vi "TEST_ASIC_SUMnADDS.vi"(0 "Instrument VISA in":T1={"AWG VISA"="generadorpulsos", "Oscilloscope  VISA "="Oscilloscope", "Integration Board IP"="172.16.7.43", "connection ID"=refnum, "report out"=refnum, "report file path"=path "C:/Documents and Settings/CTA_LAB01/Desktop/L0_Asic/L0 Asic Test Data"}, 2 "Serial number":string="SN018", 5 "quantity":i32=3, 7 "Cycles Burst":i32=10000, 9 "L1 Address":i32=17, 11 "error in":errorcluster, 12 "channel array":i32[](array[numeric])=[0, 1, 2, 3, 4, 5, 6]) -> (4 "Instrument VISA out":T1={"AWG VISA"="", "Oscilloscope  VISA "="", "Integration Board IP"="", "connection ID"=refnum, "report out"=refnum, "report file path"=path "C:/Documents and Settings/CTA_LAB01/Desktop/L0_Asic/L0 Asic Test Data"}, 15 "error out":errorcluster={"status"=TRUE, "code"=63, "source"="TCP Open Connection in Test2_3b_ASIC_mezzanine.vi->test_sum_mezzanine_ASIC.vi"})   [LabVIEW 2009]
uses:
  <vilib>/Utility/NIReport.llb/NI_report.lvclass
  <vilib>/Utility/NIReport.llb/HTML/NI_HTML.lvclass
  <instrlib>/Agilent 81150/Agilent 81150.lvlib
  <instrlib>/Agilent 8000 Series/Agilent 8000 Series.lvlib
panel:
  out "NChannels":i32
  out "Array":i32[](array[numeric])=[0, 2, 3]
  out "Filename Out":path
  out "points quantity":dbl=138.0
  out "appended array":dbl[](array[numeric])=[0.05, 11.0, 0.0, 63.0, 1.0, 9.99999e+37, 9.99999e+37, 2.068e-09, 3.4e-11, 9.99999e+37, 9.99999e+37, 9.99999e+37, 9.99999e+37, 9.99999e+37, 9.99999e+37, 138.0]
  out "read buffer 3":string="V amptd(1),9.99999E+37,9.99999E+37,9.99999E+37,9.99999E+37,9.99999E+37,1.38E+02,+ width(1),2.06E-09,1.99E-09,2.19E-09,2.068E-09,3.4E-11,1.38E+02,V amptd(f2),9.99999E+37,9.99999E+37,9.99999E+37,9.99999E+37,9.99999E+37,1.38E+02,+ width(f2),9.99999E+37,9.99999E+37,9.99999E+37,9.99999E+37,9.99999E+37,3.5E+01,Time(1-f2),9.99999E+37,9.99999E+37,9.99999E+37,9.99999E+37,9.99999E+37,1.00E+02\n"
  in  "Quantity of \nMeasurements":u32=50
  in  "Voltage":dbl[](array[numeric])=[0.05, 0.2]
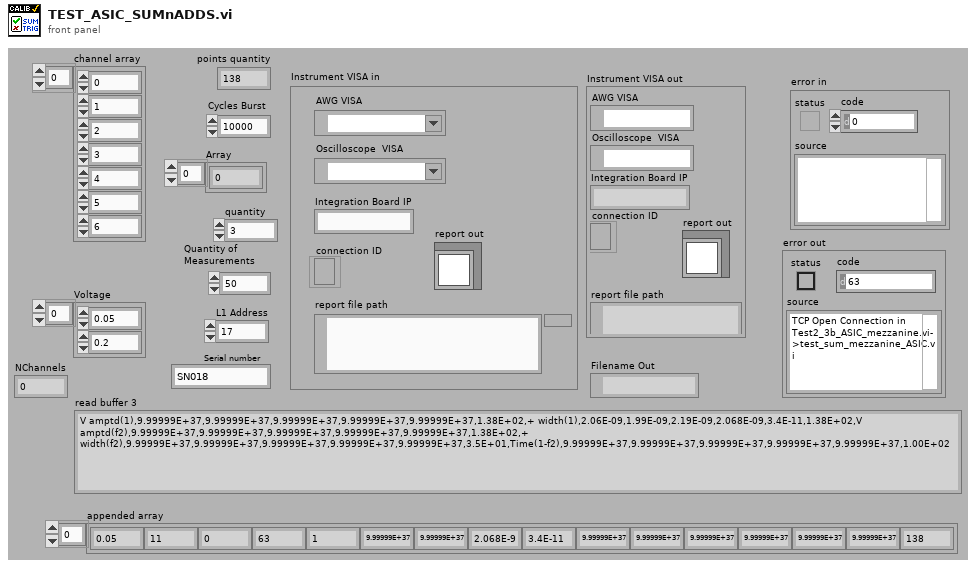
[diagram p1: front panel]
types:
  T1 = cluster{"AWG VISA":refnum<visa-resource-name>, "Oscilloscope  VISA ":refnum<visa-resource-name>, "Integration Board IP":string, "connection ID":refnum<k5>, "report out":refnum<class "NI_report.lvclass">, "report file path":path}
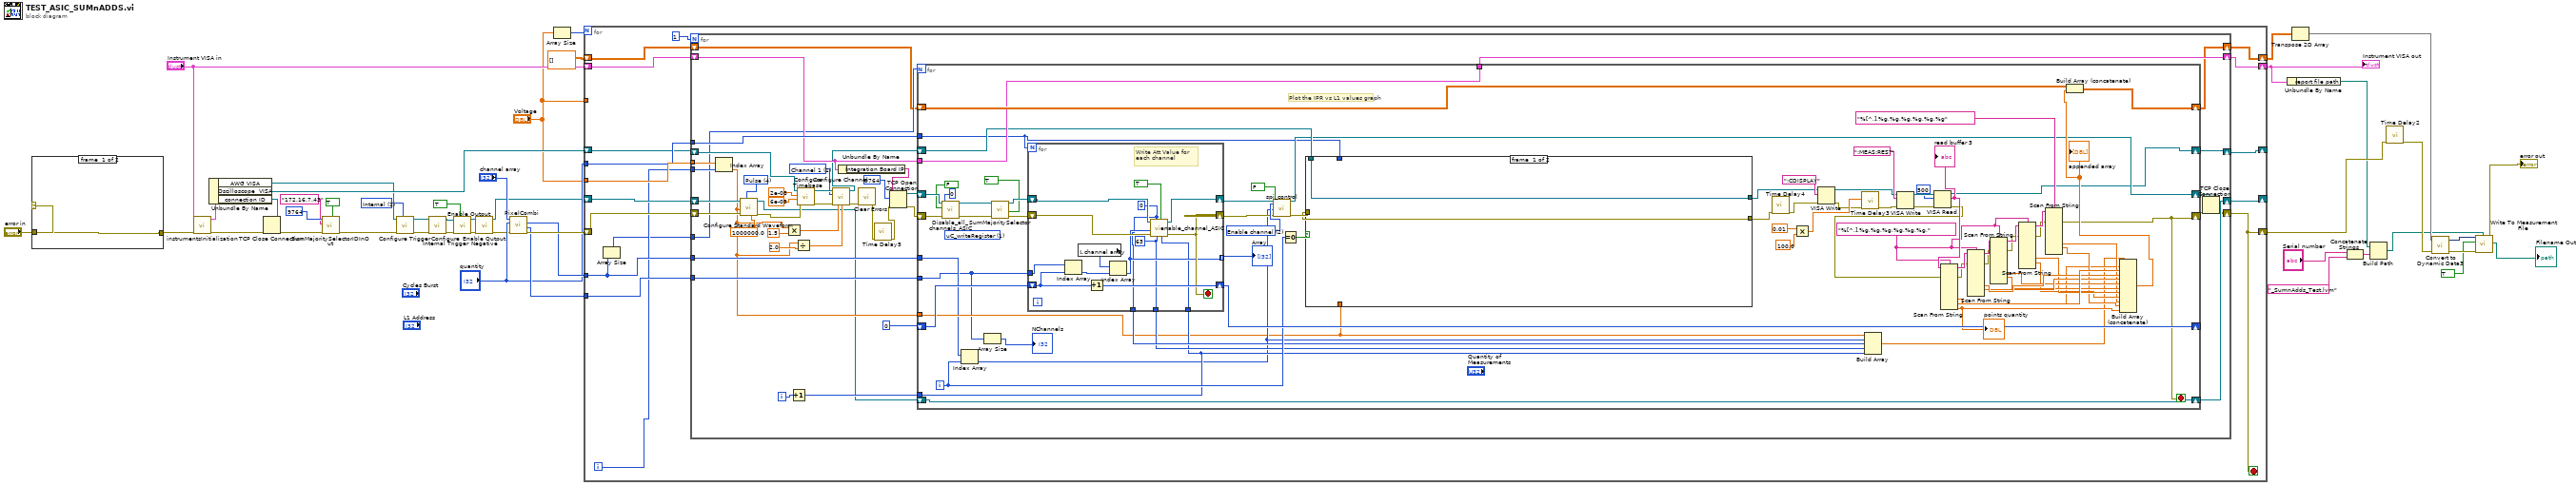
[diagram p0: block diagram]
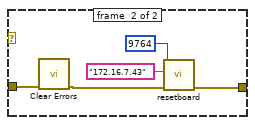
[diagram p2: hidden frame]
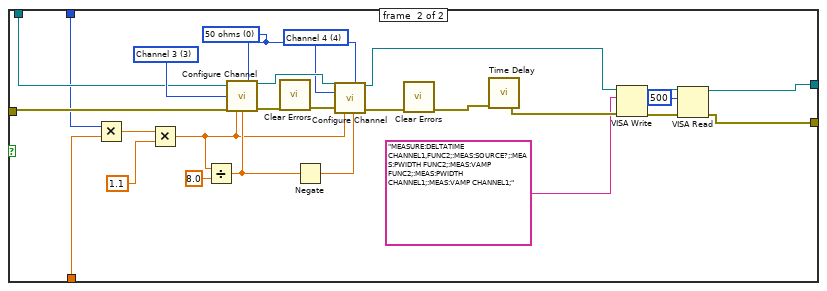
[diagram p3: hidden frame]
diagram:
  w22 = u16 1 items=["Immediate", "Internal", "External", "Software Trigger Function"] ("Trigger Source (0: Immediate)")
  n1 = case shown="Error" "error in" {
    tunnel: "error in" -> [w46 w48]
    tunnel: [w46 w51] -> w18
    frame #0 {
    }
    frame #1 {
      n2 = call <vilib>:"Clear Errors.vi"("error in (no error)"=w48) -> ("error out"=w47:errorcluster)  [unwired: 6 in]
      n3 = call "resetboard.vi"("error in (no error)"=w47, "address"="172.16.7.43", "remote port or service name"=u16 9764) -> ("error out"=w51:errorcluster)  [unwired: 7 in, 1 out]
    }
  }
  n4 = call "instrumentsInitialization.vi"("error in"=w18, "Instrument VISA in"="Instrument VISA in") -> ("error out"=w16:errorcluster, "Instrument VISA out"=w38:T1)  [unwired: 8 in]
  n5 = Unbundle By Name(w38) -> ("AWG VISA"=w25:refnum<visa-resource-name>, "Oscilloscope  VISA"=w37:refnum<visa-resource-name>, "connection ID"=w17:refnum<k5>)
  n6 = TCP Close Connection(connection ID=w17, error in (no error)=w16) -> (error out=w5:errorcluster)  [unwired: 1 in, 1 out]
  n7 = call "SumMajoritySelectorIDInOut.vi"("On Sum\nOff Majority"=TRUE ("Enable Output (T: Enable)"), "error in (no error)"=w5, "address"="172.16.7.43", "remote port or service name"=u16 9764) -> ("error out"=w1:errorcluster)  [unwired: 7 in]
  n8 = call <instrlib>:"Configure Trigger.vi"("Trigger Source (0: Immediate)"=w22, "error in (no error)"=w1, "VISA resource name"=w25) -> ("error out"=w23:errorcluster, "VISA resource name out"=w24:refnum<visa-resource-name>)  [unwired: 7 in]
  n9 = call <instrlib>:"Configure Internal Trigger.vi"("error in (no error)"=w23, "VISA resource name"=w24) -> ("error out"=w26:errorcluster, "VISA resource name out"=w27:refnum<visa-resource-name>)  [unwired: 8 in]
  n10 = call <instrlib>:"Enable Output.vi"("Enable Output (T: Enable)"=TRUE, "error in (no error)"=w26, "VISA resource name"=w27) -> ("error out"=w13:errorcluster, "VISA resource name out"=w12:refnum<visa-resource-name>)  [unwired: 7 in]
  n11 = call <instrlib>:"Enable Output Negative.vi"("error in (no error)"=w13, "VISA resource name"=w12) -> ("error out"=w14:errorcluster, "VISA resource name out"=w15:refnum<visa-resource-name>)  [unwired: 8 in]
  n12 = call "PixelCombi.vi"("error in"=w14, "quantity"="quantity", "array"="channel array") -> ("error out"=w44:errorcluster, "Channels"=w43:i32[], "Combination Array"=w42:i16[])  [unwired: 6 in]
  n13 = Array Size(array="Voltage") -> (size(s)=w39:i32)
  n14 = for {
    N: w39 -> [_]
    tunnel: w43 -> [w66]
    tunnel: w42 -> [w65]
    shift-right: [w52] -> w29
    shift-left: w44 -> [w68]
    tunnel: "Voltage" -> [w64]
    tunnel: "Voltage" -> [_]
    tunnel: "quantity" -> [w62]
    shift-right: [w57] -> w28
    shift-left: "Instrument VISA in" -> [w60]
    shift-right: [w56] -> w32
    shift-left: dbl[][] [] -> [w58]
    shift-right: [w53] -> _
    shift-left: w15 -> [w67]
    shift-right: [w54] -> _
    shift-left: w37 -> [w61]
    i -> [w63]
    stop <- w52 stop-if-true
    n15 = Array Size(array=w65) -> (size(s)=w59:i32)
    n16 = for {
      N: 1 -> [_]
      tunnel: w66 -> [w107]
      tunnel: w65 -> [w105]
      tunnel: w64 -> [w104]
      tunnel: w63 -> [w103]
      tunnel: w62 -> [w102]
      tunnel: w59 -> [w87]
      shift-right: [w77] -> w56
      shift-left: w58 -> [w80]
      shift-right: [w78] -> w57
      shift-left: w60 -> [w91]
      shift-right: [w72] -> w52
      shift-left: w68 -> [w109]
      shift-right: [w73] -> w53
      shift-left: w67 -> [w108]
      shift-right: [w75] -> w54
      shift-left: w61 -> [w98]
      i -> [w69]
      w94 = 1 items=["Channel 1"=1, "Channel 2"=2, "Channel 3"=3, "Channel 4"=4] ("Channel (1: Channel 1)")
      w111 = u16 4 items=["Sine", "Square", "Ramp Up", "Ramp Down", "Pulse", "Noise", "DC"] ("Waveform (0: Sine)")
      n17 = Index Array(array=w104, index=w103) -> (element=w79:dbl)
      n18 = call <instrlib>:"Configure Standard Waveform.vi"("Frequency (1000.0 Hz)"=1000000.0, "Waveform (0: Sine)"=w111, "error in (no error)"=w109, "Amplitude (1.0 Vpp)"=w79, "VISA resource name"=w108) -> ("error out"=w101:errorcluster, "VISA resource name out"=w74:refnum<visa-resource-name>)  [unwired: 5 in]
      n19 = Multiply(x=w79, y=1.5) -> (x*y=w93:dbl)
      n20 = Increment(x=w69) -> (x+1=w76:i32)
      n21 = Divide(x=w79, y=2.0) -> (x/y=w85:dbl)
      n22 = call <instrlib>:"Configure Timebase.vi"("error in (no error)"=w101, "Position (0.0 s)"=6e-09, "Timebase (0.005 s)"=2e-08, "VISA resource name"=w98) -> ("error out"=w100:errorcluster, "VISA resource name out"=w97:refnum<visa-resource-name>)  [unwired: 6 in]
      n23 = call <instrlib>:"Configure Channel.vi"("VISA resource name"=w97, "Channel (1: Channel 1)"=w94, "error in (no error)"=w100, "Vertical Range (2.0 V)"=w93, "Vertical Offset (0.0 V)"=w85) -> ("VISA resource name out"=w84:refnum<visa-resource-name>, "error out"=w99:errorcluster)  [unwired: 9 in]
      n24 = Unbundle By Name(w91) -> ("Integration Board IP"=w89:string)
      n25 = call <vilib>:"Clear Errors.vi"("error in (no error)"=w99) -> ("error out"=w71:errorcluster)  [unwired: 6 in]
      n26 = call "Time Delay5"("error in (no error)"=w71) -> ("error out"=w70:errorcluster)  [unwired: 10 in]
      n27 = TCP Open Connection(address=w89, remote port or service name=u16 9764, error in (no error)=w70) -> (connection ID=w81:refnum<k5>, error out=w90:errorcluster)  [unwired: 2 in]
      n28 = for {
        N: w87 -> [_]
        tunnel: w105 -> [w115]
        tunnel: w107 -> [w113]
        shift-right: [w185] -> _
        shift-left: i16 0 ("element") -> [w186]
        shift-right: [w135] -> w83
        shift-left: w90 -> [w181]
        tunnel: w91 -> [w176]
        tunnel: w102 -> [w112]
        tunnel: [w176] -> w78
        shift-right: [w182] -> w77
        shift-left: w80 -> [w183]
        shift-right: [w136] -> w82
        shift-left: w81 -> [w134]
        tunnel: w79 -> [w116]
        tunnel: w76 -> [w129]
        shift-right: [w128] -> w75
        shift-left: w84 -> [w174]
        shift-right: [w127] -> w73
        shift-left: w74 -> [w127]
        i -> [w172]
        stop <- w135 stop-if-true
        w157 = "%[^,],%g,%g,%g,%g,%g,%g," ("format string")
        w180 = u16 2 items=["Attenuation", "Clipping", "Enable channel", "Delay line", "ASIC"] ("Device")
        (unwired) u16 1 items=["sendCommand"=9, "FPGA_writeRegister"=3, "FPGA_readRegister"=2, "uC_writeRegister"=1, "uC_readRegister"=0] ("Action")
        # "Plot the IPR vs L1 values graph"
        n29 = call "Disable_all_channels_ASIC.vi"("error in"=w181, "id_in"=0 ("Data"), "Clip_en_b"=FALSE, "connection ID"=w134) -> ("error out"=w120:errorcluster, "connection ID out"=w121:refnum<k5>)  [unwired: 5 in, 1 out]
        n30 = Index Array(array=w115, index=w172) -> (element=w117:i16)
        n31 = Array Size(array=w113) -> (size(s)=→"NChannels":i32)
        n32 = call "SumMajoritySelector.vi"("On Sum\nOff Majority"=TRUE ("Clip_en_b"), "error in (no error)"=w120, "connection ID"=w121) -> ("error out"=w119:errorcluster, "connection ID out"=w122:refnum<k5>)  [unwired: 5 in]
        n33 = for {
          N: w112 -> [_]
          shift-right: [w227] -> w185
          shift-left: w186 -> [w228]
          tunnel: w113 -> [w226]
          shift-right: [w223] -> w178
          shift-left: w119 -> [w222]
          shift-right: [w220] -> w177
          shift-left: w122 -> [w221]
          tunnel: [w219] -> w123 mode=indexing
          tunnel: [w218] -> w132
          tunnel: [w217] -> w131
          tunnel: w129 -> [w216]
          stop <- w223 stop-if-true
          w218 = u32 0 ("Att gain")
          w217 = u32 63 ("Ib_clipVb")
          # "Write Att Value for each channel"
          n34 = Index Array(array=w226, index=w228) -> (element=w224:i32)
          n35 = local read "channel array"() -> (w225:i32[])
          n36 = Increment(x=w228) -> (x+1=w227:i16)
          n37 = Index Array(array=w225, index=w224) -> (element=w219:i32)
          n38 = call "enable_channel_ASIC.vi"("Clip_sel_b"=w216, "maj/sum"=TRUE, "Ib_clipVb"=w217, "Att gain"=w218, "error in"=w222, "Channel"=w219, "connection ID"=w221) -> ("error out"=w223:errorcluster, "connection ID out"=w220:refnum<k5>)  [unwired: 2 in, 1 out]
        }
        "Array" <- w123
        n39 = call "spi_control.vi"("connection ID"=w177, "Device"=w180, "Read/#write"=FALSE, "Data"=w117, "error out 3"=w178) -> ("connection ID out"=w136:refnum<k5>, "error out 2"=w175:errorcluster)  [unwired: 7 in, 6 out]
        n40 = Equal To 0?(x=w172) -> (x = 0?=w173:bool)
        n41 = case shown="True" w173 {
          tunnel: [w188 w201] -> w124
          tunnel: w175 -> [w188 w196]
          tunnel: w174 -> [w187 w197]
          tunnel: [w187 w207] -> w139
          tunnel: w116 -> [_ w192]
          tunnel: w112 -> [_ w193]
          frame #0 {
          }
          frame #1 {
            w208 = u32 0 items=["50 ohms", "1 Mohms"] ("Input Impedance (1: 1 Mohms)")
            w200 = 3 items=["Channel 1"=1, "Channel 2"=2, "Channel 3"=3, "Channel 4"=4] ("Channel (1: Channel 1)")
            w199 = 4 items=["Channel 1"=1, "Channel 2"=2, "Channel 3"=3, "Channel 4"=4] ("Channel (1: Channel 1)")
            n42 = Multiply(x=w193, y=w192) -> (x*y=w191:dbl)
            n43 = Multiply(x=w191, y=1.1) -> (x*y=w189:dbl)
            n44 = Divide(x=w189, y=8.0) -> (x/y=w194:dbl)
            n45 = call <instrlib>:"Configure Channel.vi"("VISA resource name"=w197, "Input Impedance (1: 1 Mohms)"=w208, "Channel (1: Channel 1)"=w200, "error in (no error)"=w196, "Vertical Range (2.0 V)"=w189, "Vertical Offset (0.0 V)"=w194) -> ("VISA resource name out"=w212:refnum<visa-resource-name>, "error out"=w214:errorcluster)  [unwired: 8 in]
            n46 = call <vilib>:"Clear Errors.vi"("error in (no error)"=w214) -> ("error out"=w206:errorcluster)  [unwired: 6 in]
            n47 = Negate(x=w194) -> (-x=w198:dbl)
            n48 = call <instrlib>:"Configure Channel.vi"("VISA resource name"=w212, "Input Impedance (1: 1 Mohms)"=w208, "Channel (1: Channel 1)"=w199, "error in (no error)"=w206, "Vertical Range (2.0 V)"=w189, "Vertical Offset (0.0 V)"=w198) -> ("VISA resource name out"=w204:refnum<visa-resource-name>, "error out"=w213:errorcluster)  [unwired: 8 in]
            n49 = call <vilib>:"Clear Errors.vi"("error in (no error)"=w213) -> ("error out"=w205:errorcluster)  [unwired: 6 in]
            n50 = call "Time Delay"("error in (no error)"=w205) -> ("error out"=w203:errorcluster)  [unwired: 10 in]
            n51 = VISA Write(VISA resource name=w204, write buffer="MEASURE:DELTATIME CHANNEL1,FUNC2;:MEAS:SOURCE?;:MEAS:PWIDTH FUNC2;:MEAS:VAMP FUNC2;:MEAS:PWIDTH CHANNEL1;:MEAS:VAMP CHANNEL1;", error in (no error)=w203) -> (VISA resource name out=w211:refnum<visa-resource-name>, error out=w210:errorcluster)  [unwired: 1 out]
            n52 = VISA Read(VISA resource name=w211, byte count=u32 500, error in (no error)=w210) -> (VISA resource name out=w207:refnum<visa-resource-name>, error out=w201:errorcluster)  [unwired: 2 out]
          }
        }
        n53 = call "Time Delay4"("error in (no error)"=w124) -> ("error out"=w125:errorcluster)  [unwired: 10 in]
        n54 = Multiply(x=0.01, y=100.0) -> (x*y=w164:dbl)
        n55 = VISA Write(VISA resource name=w139, write buffer=":CDISPLAY", error in (no error)=w125) -> (VISA resource name out=w142:refnum<visa-resource-name>, error out=w140:errorcluster)  [unwired: 1 out]
        n56 = call "Time Delay3"("error in (no error)"=w140, "Delay Time (s)"=w164) -> ("error out"=w163:errorcluster)  [unwired: 9 in]
        n57 = Build Array(w116, w117, w132, w131, w129) -> (w130:dbl[])
        n58 = VISA Write(VISA resource name=w142, write buffer=":MEAS:RES?", error in (no error)=w163) -> (VISA resource name out=w171:refnum<visa-resource-name>, error out=w170:errorcluster)  [unwired: 1 out]
        n59 = VISA Read(VISA resource name=w171, byte count=u32 500, error in (no error)=w170) -> (VISA resource name out=w128:refnum<visa-resource-name>, read buffer=w167:string, error out=w147:errorcluster)  [unwired: 1 out]
        "read buffer 3" <- w167
        n60 = Scan From String(format string=w157, input string=w167, error in=w147) -> (remaining string=w161:string, error out=w143:errorcluster, output 5=w133:dbl, output 6=w162:dbl, output 7=w148:dbl)  [unwired: 12 in, 1 out]
        "points quantity" <- w148
        n61 = Scan From String(format string=w157, input string=w161, error in=w143) -> (remaining string=w158:string, error out=w144:errorcluster, output 5=w155:dbl, output 6=w154:dbl)  [unwired: 13 in, 1 out]
        n62 = Scan From String(format string=w157, input string=w158, error in=w144) -> (remaining string=w159:string, error out=w145:errorcluster, output 5=w153:dbl, output 6=w152:dbl)  [unwired: 13 in, 1 out]
        n63 = Scan From String(format string=w157, input string=w159, error in=w145) -> (remaining string=w160:string, error out=w146:errorcluster, output 5=w151:dbl, output 6=w150:dbl)  [unwired: 13 in, 1 out]
        n64 = Scan From String(format string="%[^,],%g,%g,%g,%g,%g,%g", input string=w160, error in=w146) -> (error out=w135:errorcluster, output 5=w138:dbl, output 6=w149:dbl)  [unwired: 13 in, 2 out]
        n65 = Build Array (concatenate)(w130, w133, w162, w155, w154, w153, w152, w151, w150, w138, w149, w148) -> (w137:dbl[])
        "appended array" <- w137
        n66 = Build Array (concatenate)(w183, w137) -> (w182:dbl[][])
      }
      n67 = TCP Close Connection(connection ID=w82, error in (no error)=w83) -> (error out=w72:errorcluster)  [unwired: 1 in, 1 out]
    }
  }
  "Instrument VISA out" <- w28
  n68 = Unbundle By Name(w28) -> ("report file path"=w7:path)
  n69 = Transpose 2D Array(2D array=w32) -> (transposed array=w20:dbl[][])
  n70 = Concatenate Strings("Serial number", "_SumnAdds_Test.lvm" ("name or relative path")) -> (w35:string)
  n71 = Build Path(base path=w7, name or relative path=w35) -> (appended path=w6:path)
  n72 = call "Time Delay2"("error in (no error)"=w29) -> ("error out"=w40:errorcluster)  [unwired: 10 in]
  n73 = call "Convert to Dynamic Data3"("2D Array"=w20) -> ("Dynamic Data Type"=w21:dynamicdata)  [unwired: 3 in]
  n74 = call "Write To Measurement File"("Signals"=w21, "Enable"=TRUE, "error in (no error)"=w40, "Filename"=w6) -> ("Filename Out"=→"Filename Out":path, "error out"=→"error out":errorcluster)  [unwired: 13 in, 1 out]
